vi "TH_crossing.vi"(0 "NewData":i16[][](array[numeric]), 1 "Threshold":i32, 2 "FileMonChan":i32, 3 "MeanIn":dbl, 4 "MeanSmoothFac":dbl=0.01) -> (5 "Crossing?":bool, 6 "MeanOut":dbl)   [LabVIEW 2018]
uses:
  D:/LabVIEW/LabVIEWProjects/dlcTAF/dlcTAF1.1/SubVIs/64bitC_code/TH_Crossing_C/bin/Debug/TH_Crossing_C.dll
panel:
  in  "Temp":i32
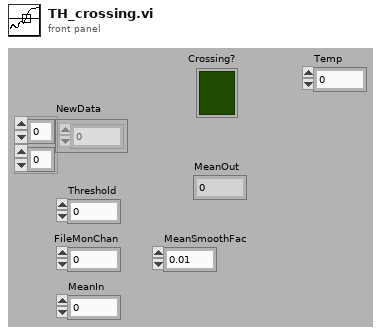
[diagram p1: front panel]
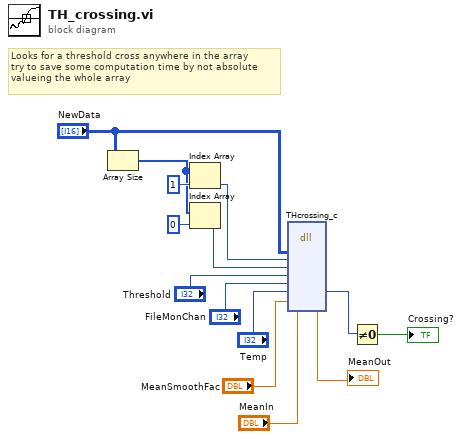
[diagram p0: block diagram]
diagram:
  # "Looks for a threshold cross anywhere in the array\ntry to save some computation time by not absolute\nvalueing the whole array"
  n1 = Array Size(array="NewData") -> (size(s)=w11:i32[])
  n2 = Index Array(array=w11, index=1) -> (element=w9:i32)
  n3 = Index Array(array=w11, index=0) -> (element=w8:i32)
  n4 = dll-call lib="D:/LabVIEW/LabVIEWProjects/dlcTAF/dlcTAF1.1/SubVIs/64bitC_code/TH_Crossing_C/bin/Debug/TH_Crossing_C.dll" fn="THcrossing_c"("NewData"="NewData", "Nnew"=w9, "Nchan"=w8, "TH"="Threshold", "MonChan"="FileMonChan", "Crossing"="Temp", "MeanSmoothFac"="MeanSmoothFac", "Mean"="MeanIn") -> ("Crossing"=w4:i32, "Mean"=→"MeanOut":dbl)  [unwired: 10 in, 2 out]
  n5 = Not Equal To 0?(x=w4) -> (x != 0?=→"Crossing?":bool)
